vi "easy stream stop.vi"(8 "error in":errorcluster, 11 "Handle In":i32) -> (0 "error out":errorcluster, 1 "Error Message":string, 3 "Handle Out":i32)   [LabVIEW 2020]
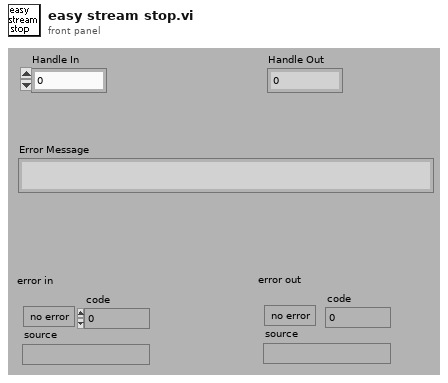
[diagram p1: front panel]
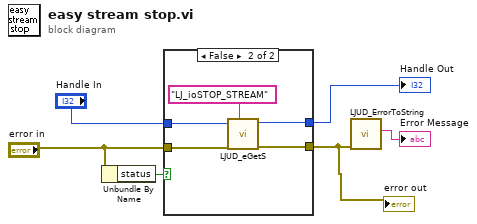
[diagram p0: block diagram]
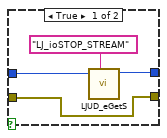
[diagram p2: hidden frame]
diagram:
  n1 = Unbundle By Name("error in") -> ("status"=w6:bool)
  n2 = case shown="False" w6 {
    tunnel: [w9 w14] -> w1
    tunnel: "error in" -> [w9 w13]
    tunnel: "Handle In" -> [w8 w12]
    tunnel: [w7 w11] -> w2
    frame True {
      n3 = call "LJUD_eGetS.vi"("IOType"="LJ_ioSTOP_STREAM", "Handle In"=w8) -> ("Handle Out"=w7:i32)  [unwired: 7 in, 2 out]
    }
    frame False {
      n4 = call "LJUD_eGetS.vi"("IOType"="LJ_ioSTOP_STREAM", "error in"=w13, "Handle In"=w12) -> ("error out"=w14:errorcluster, "Handle Out"=w11:i32)  [unwired: 6 in, 1 out]
    }
  }
  "Handle Out" <- w2
  "error out" <- w1
  n5 = call "LJUD_ErrorToString.vi"("error in"=w1) -> ("String"=→"Error Message":string)  [unwired: 10 in]
